vi "stringArray.vi"(3 "Array Length":i32=-1, 4 "Array":string[](array[string]), 5 "msg in":string) -> (2 "msg out":string)   [LabVIEW 2015]
doc: "Flattens a string array into a message"
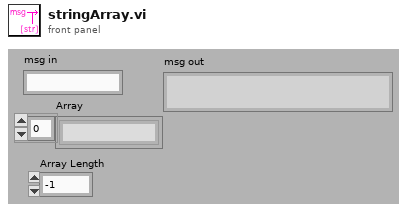
[diagram p1: front panel]
types:
  T1 = enum16{"big-endian, network order", "native, host order", "little-endian"}
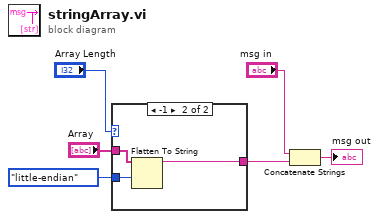
[diagram p0: block diagram]
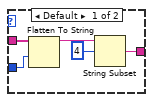
[diagram p2: hidden frame]
diagram:
  n1 = case shown="-1" "Array Length" {
    tunnel: T1."little-endian" ("byte order (0:big-endian, network order)") -> [w10 w14]
    tunnel: [w8 w13] -> w5
    tunnel: "Array" -> [w11 w12]
    frame Default {
      n2 = Flatten To String(anything=w11, byte order (0:big-endian, network order)=w10) -> (data string=w9:string)  [unwired: 2 in, 2 out]
      n3 = String Subset(string=w9, offset (0)=4 ("length (rest)")) -> (substring=w8:string)  [unwired: 1 in]
    }
    frame -1 {
      n4 = Flatten To String(anything=w12, byte order (0:big-endian, network order)=w14) -> (data string=w13:string)  [unwired: 2 in, 2 out]
    }
  }
  n5 = Concatenate Strings("msg in", w5) -> (→"msg out":string)
